vi "Built electrical data file.vi"() -> (3 "Spreadsheet string out":string)   [LabVIEW 2013]
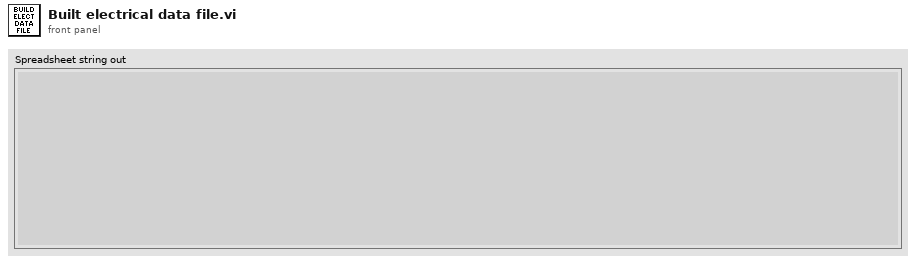
[diagram p1: front panel]
types:
  T1 = typedef "electrical.ctl" = cluster{"date/time string":string, "Electrical Data Labels":string[], "Electrical Data":string[], "Waveform Graph":waveform(dbl)[]}
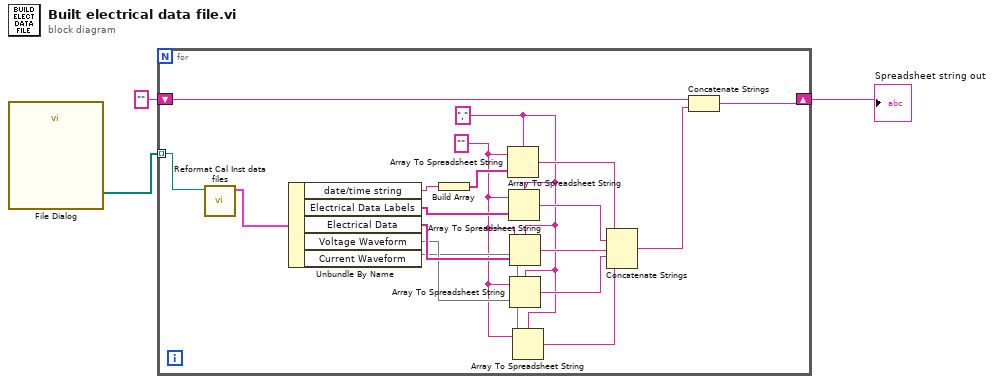
[diagram p0: block diagram]
diagram:
  n1 = call "File Dialog"() -> ("selected paths"=w3:path[])  [unwired: 12 in, 3 out]
  n2 = for {
    tunnel: w3 -> [w21] mode=indexing
    shift-right: [w11] -> w1
    shift-left: "" -> [w10]
    w5 = "" ("format string")
    w4 = "," ("delimiter (Tab)")
    n3 = call "Reformat Cal Inst data files.vi"("file path (dialog if empty)"=w21) -> ("Electrical Data"=w20:T1)  [unwired: 10 in]
    n4 = Unbundle By Name(w20) -> ("date/time string"=w7:string, "Electrical Data Labels"=w19:string[], "Electrical Data"=w18:string[], "Voltage Waveform"=w17, "Current Waveform"=w16)
    n5 = Build Array(w7) -> (w6:string[])
    n6 = Array To Spreadsheet String(delimiter (Tab)=w4, array=w6, 3:w5) -> (spreadsheet string=w8:string)
    n7 = Array To Spreadsheet String(delimiter (Tab)=w4, array=w19, 3:w5) -> (spreadsheet string=w15:string)
    n8 = Array To Spreadsheet String(delimiter (Tab)=w4, array=w18, 3:w5) -> (spreadsheet string=w14:string)
    n9 = Array To Spreadsheet String(delimiter (Tab)=w4, array=w17, 3:w5) -> (spreadsheet string=w13:string)
    n10 = Array To Spreadsheet String(delimiter (Tab)=w4, array=w16, 3:w5) -> (spreadsheet string=w12:string)
    n11 = Concatenate Strings(w8, w15, w14, w13, w12) -> (w9:string)
    n12 = Concatenate Strings(w10, w9) -> (w11:string)
  }
  "Spreadsheet string out" <- w1
